vi "Recognise_String Data to 2D Array.vi"(8 "error in (no error)":errorcluster, 10 "Max Possibility":i32, 11 "Detected Licence Plates as String":string) -> (0 "error out":errorcluster, 3 "Processed Recognise Data":string[][](array[string]))   [LabVIEW 2014, in "OpenALPR in LabView.lvlib"]
doc: "Process the data, so we can read in the recognise data in labview as a 2d Array. Get in the Recognised data as String and return it as a LabVIEW 2D Array. You can save this data to files or use it in your application as a normal Array.\n\nUse this SubVI for Data conbersation for your own application."
uses:
  OpenALPR in LabView.lvlib
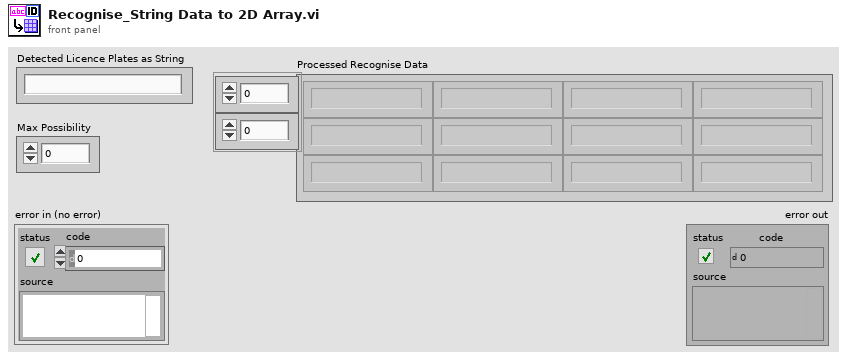
[diagram p1: front panel]
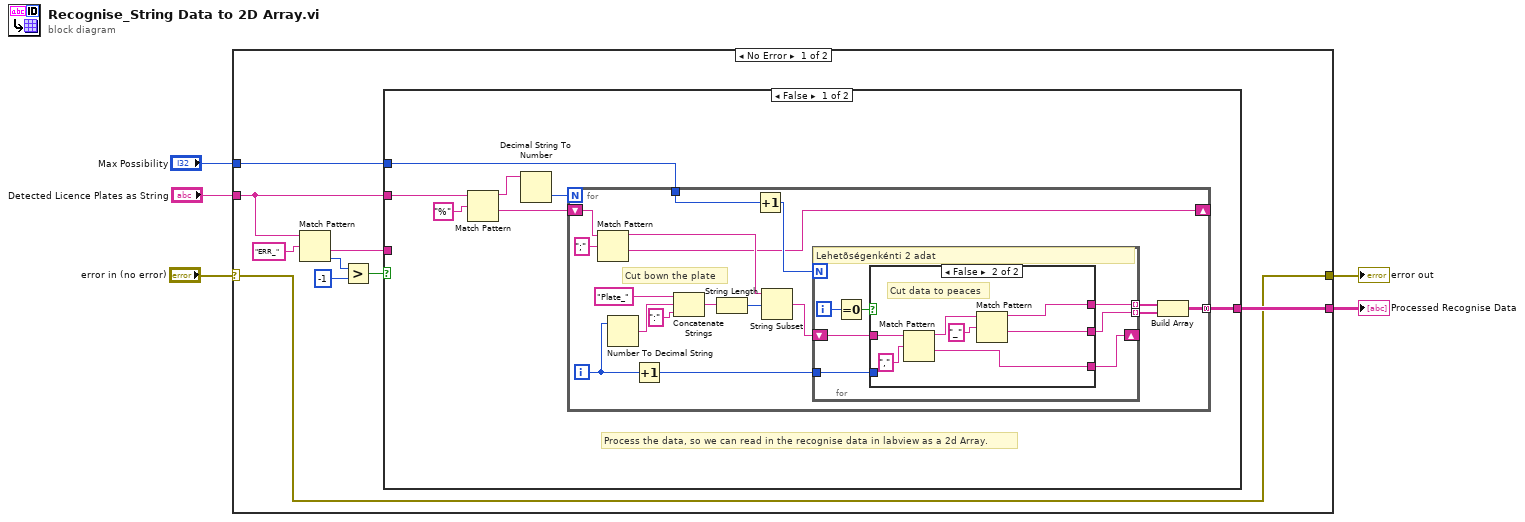
[diagram p0: block diagram]
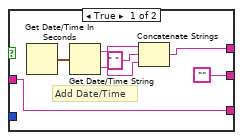
[diagram p2: hidden frame]
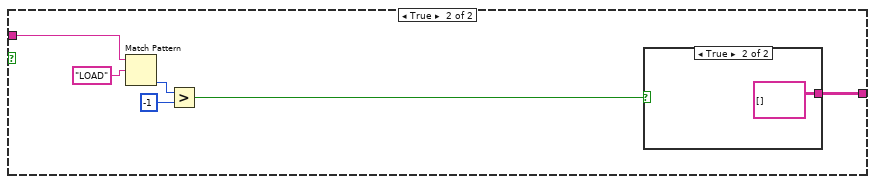
[diagram p3: hidden frame]
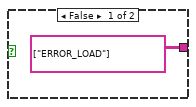
[diagram p4: hidden frame]
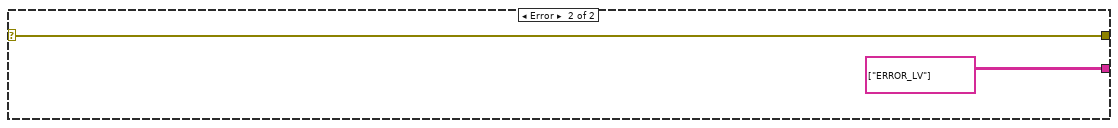
[diagram p5: hidden frame]
diagram:
  n1 = case shown="No Error" "error in (no error)" {
    selector: "error in (no error)" -> [w6 w68]
    tunnel: "Max Possibility" -> [w14 _]
    tunnel: [w13 string[][] [["ERROR_LV"]]] -> w4
    tunnel: "Detected Licence Plates as String" -> [w11 _]
    tunnel: [w6 w68] -> w1
    frame No Error {
      n2 = Match Pattern(string=w11, regular expression="ERR_" ("search string")) -> (after substring=w7:string, offset past match=w10:i32)  [unwired: 1 in, 2 out]
      n3 = Greater?(x=w10, y=-1) -> (0:w8:bool)
      n4 = case shown="False" w8 {
        tunnel: w14 -> [w21 _]
        tunnel: [w20 w65] -> w13
        tunnel: w11 -> [w15 _]
        tunnel: w7 -> [_ w60]
        frame False {
          # "Process the data, so we can read in the recognise data in labview as a 2d Array."
          n5 = Match Pattern(string=w15, regular expression="%" ("search string")) -> (before substring=w17:string, after substring=w16:string)  [unwired: 1 in, 2 out]
          n6 = Decimal String To Number(string=w17) -> (number=w18:i32)  [unwired: 2 in, 1 out]
          n7 = for {
            N: w18 -> [_]
            tunnel: [w23] -> w20 mode=concatenating
            shift-right: [w26] -> _
            shift-left: w16 -> [w30]
            tunnel: w21 -> [w22]
            i -> [w28]
            # "Cut bown the plate"
            n8 = Match Pattern(string=w30, regular expression=";") -> (before substring=w27:string, after substring=w26:string)  [unwired: 1 in, 2 out]
            n9 = Number To Decimal String(number=w28) -> (decimal integer string=w37:string)  [unwired: 1 in]
            n10 = Increment(x=w28) -> (x+1=w29:i32)
            n11 = Concatenate Strings("Plate_" ("string"), w37, ":" ("string")) -> (w35:string)
            n12 = String Length(string=w35) -> (length=w34:i32)
            n13 = Increment(x=w22) -> (x+1=w31:i32)
            n14 = String Subset(string=w27, offset (0)=w34) -> (substring=w32:string)  [unwired: 1 in]
            n15 = for {
              N: w31 -> [_]
              shift-right: [w44] -> _
              shift-left: w32 -> [w45]
              tunnel: w29 -> [w41]
              tunnel: [w40] -> w25 mode=indexing
              tunnel: [w39] -> w24 mode=indexing
              i -> [w42]
              # "Lehetõségenkénti 2 adat"
              n16 = Equal To 0?(x=w42) -> (x = 0?=w43:bool)
              n17 = case shown="False" w43 {
                tunnel: w45 -> [w52 w58]
                tunnel: [w52 w57] -> w44
                tunnel: [w48 w54] -> w40
                tunnel: ["" w53] -> w39
                tunnel: w41 -> [_ _]
                frame True {
                  # "Add Date/Time"
                  n18 = Get Date/Time In Seconds() -> (seconds since 1Jan1904=w50:timestamp)
                  n19 = Get Date/Time String(seconds (now)=w50) -> (date string=w47:string, time string=w46:string)  [unwired: 2 in]
                  n20 = Concatenate Strings(w47, " " ("string"), w46) -> (w48:string)
                }
                frame False {
                  # "Cut data to peaces"
                  n21 = Match Pattern(string=w58, regular expression=",") -> (before substring=w55:string, after substring=w57:string)  [unwired: 1 in, 2 out]
                  n22 = Match Pattern(string=w55, regular expression="_" ("search string")) -> (before substring=w54:string, after substring=w53:string)  [unwired: 1 in, 2 out]
                }
              }
            }
            n23 = Build Array(w25, w24) -> (w23:string[][])
          }
        }
        frame True {
          n24 = Match Pattern(string=w60, regular expression="LOAD" ("search string")) -> (offset past match=w63:i32)  [unwired: 1 in, 3 out]
          n25 = Greater?(x=w63, y=-1) -> (0:w61:bool)
          n26 = case shown="True" w61 {
            tunnel: [string[][] [["ERROR_LOAD"]] string[][] []] -> w65
            frame False {
            }
            frame True {
            }
          }
        }
      }
    }
    frame Error {
    }
  }
  "Processed Recognise Data" <- w4
  "error out" <- w1
